vi "Main.vi"() -> ()   [LabVIEW 2019]
doc: "Use this template to build a simple state machine design pattern. Each state executes code and determines which state to transition to."
uses:
  <vilib>/Utility/file.llb/Write Delimited Spreadsheet (string).vi
panel:
  out "error out 2":errorcluster
  out "error out":errorcluster
  in  "Focus":bool
  in  "Start":bool
  in  "File Open":bool
  out "GPS Data":string[][](table)
  in  "Add":bool
  out "GPS Status":bool
  out "Image folder":path caption="Path"
  out "Statusbar":string="Idle"
  out "Build Version":string="Idle" caption="V"
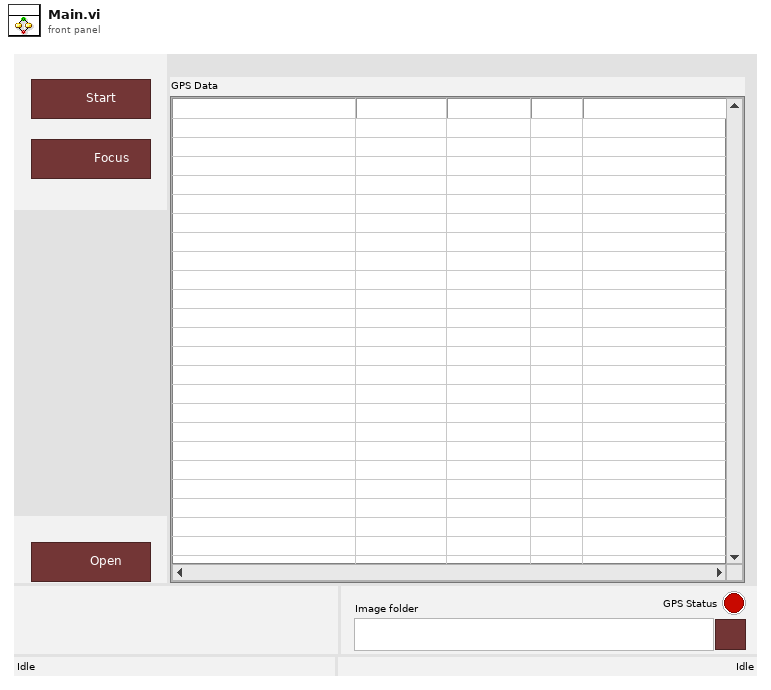
[diagram p1: front panel]
types:
  T1 = enum32{"Invalid", "Standard", "Closed", "Hidden", "Minimized", "Maximized"}
  T2 = enum32{"invalid app kind", "Development System", "Run Time System", "Student Edition", "Embedded LabVIEW", "Evaluation", "Custom"}
  T3 = typedef "System Data.ctl" = cluster{"System":cluster{"Active":bool, "Exit":bool, "Command wait":string, "Status_Time":i32, "Time_GPS":i32}, "Stepper Motor":T4, "Camera Data":T5, "Core":cluster{"Close Panel on Exit?":bool, "Current VI Reference":refnum<vi>}}
  T4 = typedef "Stepper Data.ctl" = cluster{"Connection Reference":refnum<visa-resource-name>, "Valid Connection":bool, "Speed":i32}
  T5 = typedef "Camera Data.ctl" = cluster{"Image path":path, "Filenames":string[], "Filenames queue":string[]}
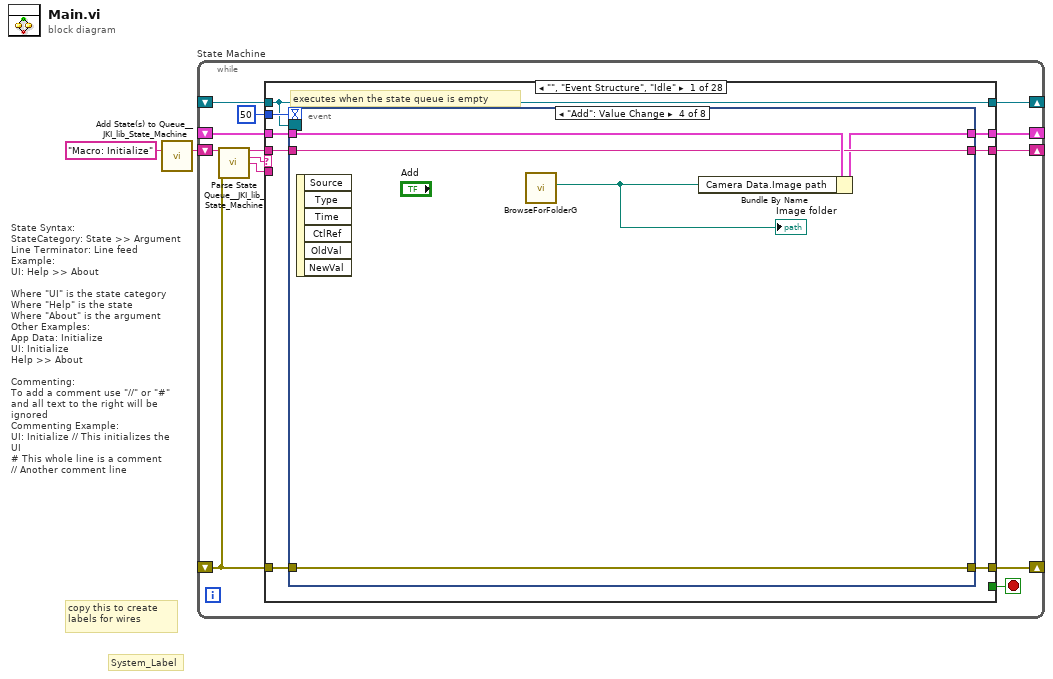
[diagram p0: block diagram]
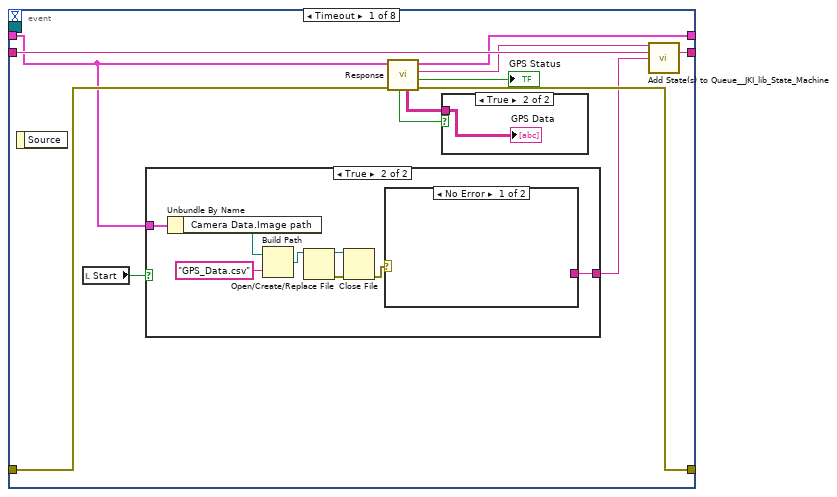
[diagram p2: hidden frame]
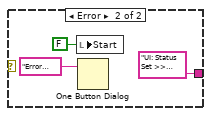
[diagram p5: hidden frame]
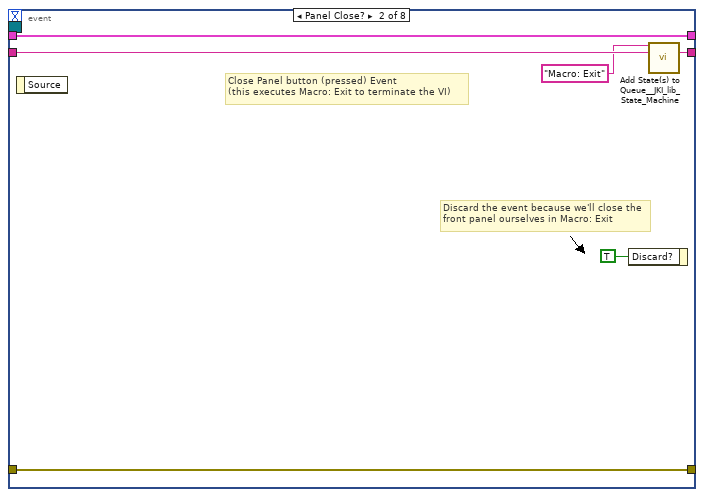
[diagram p6: hidden frame]
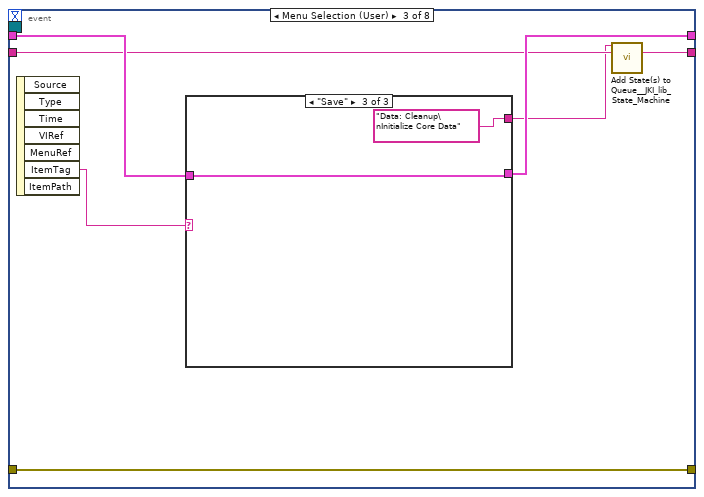
[diagram p7: hidden frame]
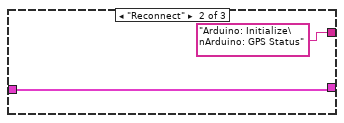
[diagram p9: hidden frame]
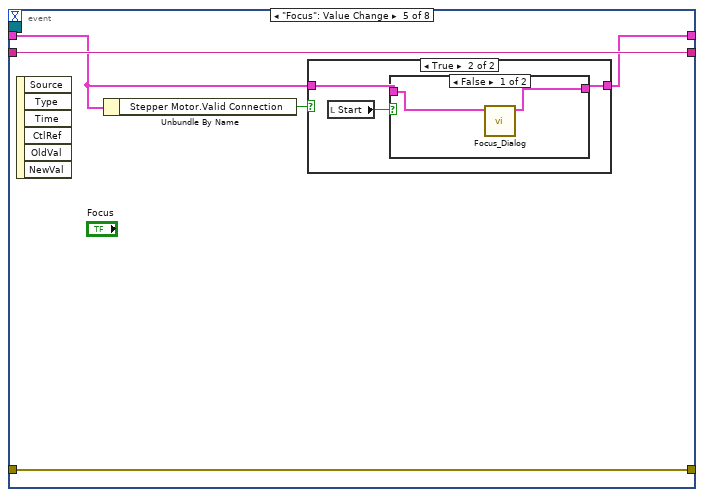
[diagram p10: hidden frame]
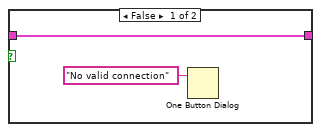
[diagram p11: hidden frame]
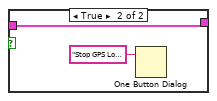
[diagram p12: hidden frame]
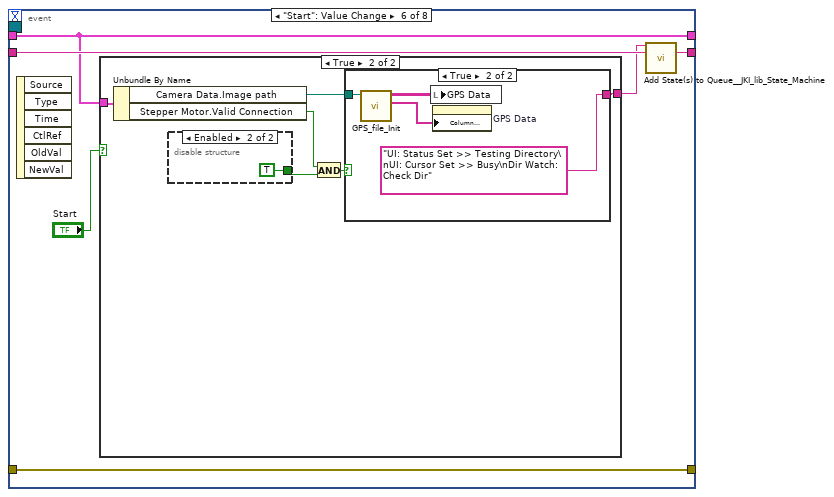
[diagram p13: hidden frame]
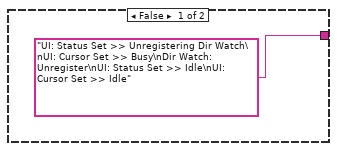
[diagram p14: hidden frame]
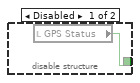
[diagram p15: hidden frame]
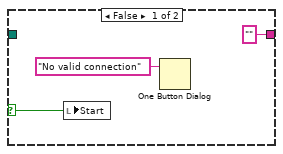
[diagram p16: hidden frame]
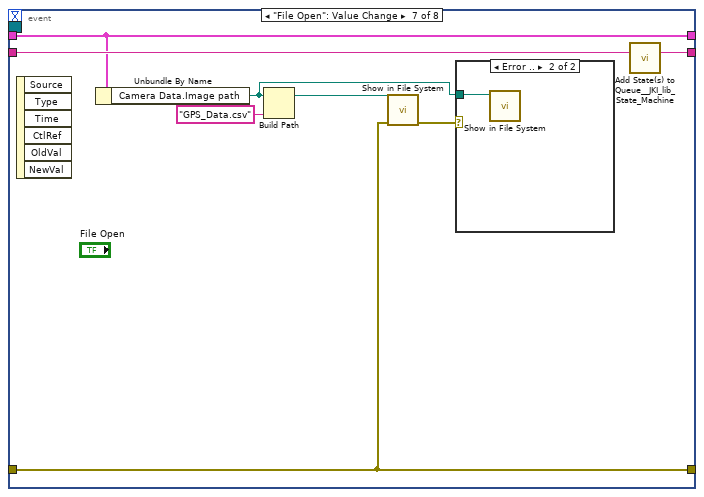
[diagram p17: hidden frame]
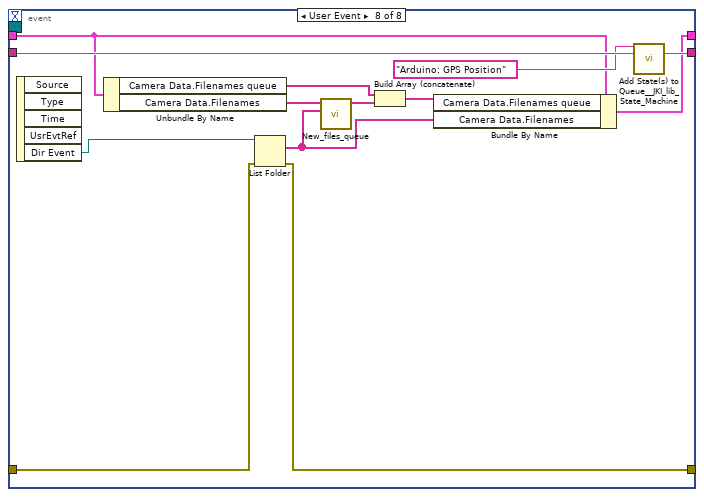
[diagram p19: hidden frame]
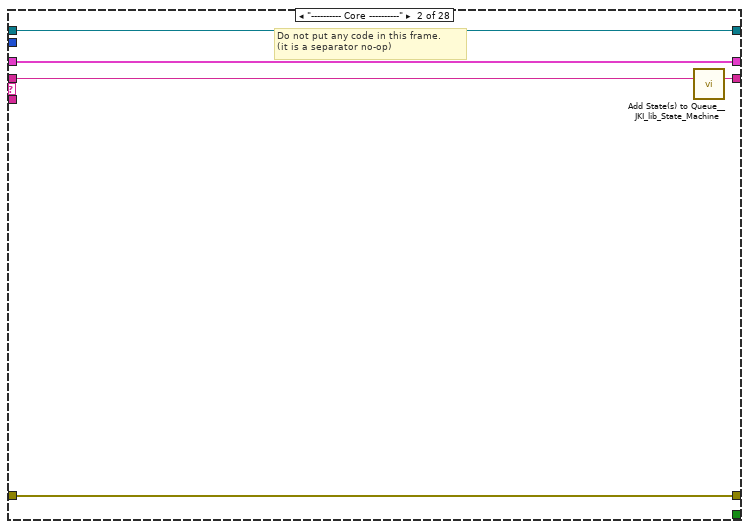
[diagram p20: hidden frame]
diagram:
  # "State Syntax:\nStateCategory: State >> Argument\nLine Terminator: Line feed\nExample:\nUI: Help >> About\n\nWhere \"UI\" is the state category\nWhere \"Help\" is the state\nWhere \"About\" is the argument\nOther Examples:\nApp Data: Initialize\nUI: Initialize\nHelp >> About\n\nCommenting:\nTo add a comment use \"//\" or \"#\" and all text to the right will be ignored\nCommenting Example:\nUI: Initialize // This initializes the UI\n# This whole line is a comment\n// Another comment line"
  # "copy this to create labels for wires"
  # "System_Label"
  n1 = call <vilib>:"Add State(s) to Queue__JKI_lib_State_Machine.vi"("State(s) in (\"\")"="Macro: Initialize") -> ("States Out"=w2:string)  [unwired: 14 in]
  n2 = while "State Machine" {
    shift-right: [w8] -> _
    shift-left: _ -> [w7]
    shift-right: [w11] -> _
    shift-left: _ -> [w5]
    shift-right: [w10] -> _
    shift-left: w2 -> [w12]
    shift-right: [w4] -> _
    shift-left: _ -> [w3]
    stop <- w9 stop-if-true
    n3 = call <vilib>:"Parse State Queue__JKI_lib_State_Machine.vi"("State Queue"=w12, "Error In (no error)"=w5) -> ("Remaining States"=w14:string, "Current State"=w15:string, "Arguments"=w13:string)  [unwired: 11 in]
    n4 = case shown="\"\", \"Event Structure\", \"Idle\"" w15 {
      selector: w15 -> [_ _ w135 _ _ _ _ _ _ _ _ _ _ _ _ _ _ _ _ _ _ _ _ _ _ _ _ _]
      tunnel: w14 -> [w23 w133 w139 w159 w168 w174 w179 w191 w198 w204 w209 w216 w223 w233 w241 w311 w317 w331 w336 w342 w349 w356 w363 w369 w376 w382 w391 w410]
      tunnel: w13 -> [_ _ _ _ _ _ _ _ _ _ _ _ w218 w229 w238 _ _ _ _ _ _ _ _ _ _ _ _ _]
      tunnel: w7 -> [w21 w130 w137 w152 w165 w172 w176 _ w192 w201 w206 w213 w221 w231 w234 w308 w314 w328 w333 w338 w346 w353 w359 w366 w374 w380 w388 w400]
      tunnel: [w20 w131 w141 w156 errorcluster {"status"=FALSE, "code"=0, "source"=""} ("error out") w171 w177 w189 w194 w200 w207 w210 w219 w228 w236 w309 w315 w329 w334 w340 w344 w350 w361 w367 w370 w379 w389 w408] -> w11
      tunnel: w5 -> [w19 w131 w140 w156 w160 w171 w177 w189 w193 w200 w207 w210 w220 w228 w239 w309 w315 w329 w334 w340 w345 w351 w361 w367 w373 w378 w389 w408]
      tunnel: [w22 w132 w138 w158 w167 w173 w178 w190 w197 w203 w208 w215 w222 w232 w240 w310 w316 w330 w335 w341 w348 w355 w362 w368 w375 w381 w390 w409] -> w10
      tunnel: [_ _ _ _ _ TRUE _ _ _ _ _ _ _ _ _ _ _ _ _ _ _ _ _ _ _ _ _ _] -> w9
      tunnel: [w18 w130 w137 w157 w163 w172 w176 w187 w192 w201 w206 w213 w221 w231 w234 w308 w314 w324 w333 w337 w343 w352 w359 w366 w371 w380 w387 w400] -> w8
      tunnel: 50 ("Timeout") -> [w17 _ _ _ _ _ _ _ _ _ _ _ _ _ _ _ _ _ _ _ _ _ _ _ _ _ _ _]
      tunnel: [w16 w129 w134 w146 w164 w170 w175 w188 w195 w202 w205 w214 w217 w230 w237 w307 w312 w322 w332 w339 w347 w354 w360 w365 w372 w377 w384 w406] -> w4
      tunnel: w3 -> [w16 w129 w134 w146 w164 w170 w175 w188 w195 w202 w205 w214 w217 w230 w237 w307 w312 w322 w332 w339 w347 w354 w360 w365 _ w377 w384 w406]
      frame "", "Event Structure", "Idle" {
        # "executes when the state queue is empty"
        n5 = event shown="[3] \"Add\": Value Change" {
          selector: w16 -> [_ _ _ _ _ _ _ _]
          dyn-events: _ -> [_ _ _ _ _ _ _ _]
          timeout: w17 -> [_ _ _ _ _ _ _ _]
          tunnel: w23 -> [w35 w53 w56 w69 w75 w89 w114 w125]
          tunnel: [w34 w52 w55 w69 w75 w88 w113 w126] -> w22
          tunnel: w21 -> [w27 w50 w58 w70 w72 w85 w112 w122]
          tunnel: [w29 w51 w60 w68 w74 w90 w107 w116] -> w20
          tunnel: w19 -> [w33 w51 w60 w68 w74 w90 w107 w127]
          tunnel: [w32 w50 w57 w67 w73 w85 w112 w120] -> w18
          event Timeout {
            n6 = event-data() -> ()  [unwired: 1 in, 1 out]
            n7 = local read "Start"() -> (w28:bool)
            n8 = case shown="True" w28 {
              tunnel: w27 -> [_ w44]
              tunnel: [_ w41] -> w26
              frame False {
              }
              frame True {
                n9 = Unbundle By Name(w44) -> ("Camera Data.Image path"=w42:path)
                n10 = Build Path(base path=w42, name or relative path="GPS_Data.csv") -> (appended path=w38:path)
                n11 = Open/Create/Replace File(file path (use dialog)=w38) -> (refnum out=w40:refnum<file>, error out=w39:errorcluster)  [unwired: 5 in, 1 out]
                n12 = Close File(refnum=w40, error in=w39) -> (error out=w37:errorcluster)  [unwired: 1 out]
                n13 = case shown="No Error" w37 {
                  tunnel: [_ "UI: Status Set >> Unregistering Dir Watch\nUI: Cursor Set >> Busy\nDir Watch: Unregister\nUI: Status Set >> Idle\nUI: Cursor Set >> Idle"] -> w41
                  frame No Error {
                  }
                  frame Error {
                    n14 = local write "Start"(FALSE ("Start")) -> ()
                    n15 = One Button Dialog(message="Error accessing GPS file\n\nClose file if open") -> ()  [unwired: 1 in, 1 out]
                  }
                }
              }
            }
            n16 = call "Response.vi"("error in"=w33, "System Data"=w27) -> ("error out"=w29:errorcluster, "GPS Status"=→"GPS Status":bool, "next state"=w31:string, "System Data out"=w32:T3, "Data"=w24:string[][], "NewData"=w25:bool)  [unwired: 4 in]
            n17 = case shown="True" w25 {
              tunnel: w24 -> [_ w36]
              frame False {
              }
              frame True {
                "GPS Data" <- w36
              }
            }
            n18 = call <vilib>:"Add State(s) to Queue__JKI_lib_State_Machine.vi"("State(s) in Front (\"\")"=w31, "State(s) in (\"\")"=w35, "State(s) at Back (\"\")"=w26) -> ("States Out"=w34:string)  [unwired: 12 in]
          }
          event Panel Close? {
            # "Discard the event because we'll close the front panel ourselves in Macro: Exit"
            # "Close Panel button (pressed) Event\n(this executes Macro: Exit to terminate the VI)"
            n19 = event-data() -> ()  [unwired: 1 in, 1 out]
            n20 = event-data("Discard?"=TRUE) -> ()  [unwired: 1 in, 1 out]
            n21 = call <vilib>:"Add State(s) to Queue__JKI_lib_State_Machine.vi"("State(s) in Front (\"\")"="Macro: Exit", "State(s) in (\"\")"=w53) -> ("States Out"=w52:string)  [unwired: 13 in]
          }
          event Menu Selection (User) {
            n22 = event-data() -> ("ItemTag"=w59:string)  [unwired: 1 in, 6 out]
            n23 = case shown="\"Save\"" w59 {
              tunnel: w58 -> [w61 w63 w65]
              tunnel: [w61 w63 w65] -> w57
              tunnel: [_ "Arduino: Initialize\nArduino: GPS Status" "Data: Cleanup\nInitialize Core Data"] -> w54
              frame "False", Default {
              }
              frame "Reconnect" {
              }
              frame "Save" {
              }
            }
            n24 = call <vilib>:"Add State(s) to Queue__JKI_lib_State_Machine.vi"("State(s) in Front (\"\")"=w54, "State(s) in (\"\")"=w56) -> ("States Out"=w55:string)  [unwired: 13 in]
          }
          event "Add": Value Change {
            n25 = event-data() -> ()  [unwired: 1 in, 6 out]
            n26 = call "BrowseForFolderG.vi"() -> ("Selected Path"=w66:path)  [unwired: 8 in, 3 out]
            "Image folder" <- w66
            n27 = Bundle By Name(cluster=w70, "Camera Data.Image path"=w66) -> (w67:T3)
          }
          event "Focus": Value Change {
            n28 = event-data() -> ()  [unwired: 1 in, 6 out]
            n29 = Unbundle By Name(w72) -> ("Stepper Motor.Valid Connection"=w71:bool)
            n30 = case shown="True" w71 {
              tunnel: [w77 w80] -> w73
              tunnel: w72 -> [w77 w79]
              frame False {
                n31 = One Button Dialog(message="No valid connection") -> ()  [unwired: 1 in, 1 out]
              }
              frame True {
                n32 = local read "Start"() -> (w78:bool)
                n33 = case shown="False" w78 {
                  tunnel: [w82 w84] -> w80
                  tunnel: w79 -> [w81 w84]
                  frame False {
                    n34 = call "Focus_Dialog.vi"("System Data"=w81) -> ("System Data out"=w82:T3)  [unwired: 10 in]
                  }
                  frame True {
                    n35 = One Button Dialog(message="Stop GPS Log before focusing") -> ()  [unwired: 1 in, 1 out]
                  }
                }
              }
            }
          }
          event "Start": Value Change {
            n36 = event-data() -> ()  [unwired: 1 in, 6 out]
            n37 = case shown="True" "Start" {
              tunnel: ["UI: Status Set >> Unregistering Dir Watch\nUI: Cursor Set >> Busy\nDir Watch: Unregister\nUI: Status Set >> Idle\nUI: Cursor Set >> Idle" w97] -> w87
              tunnel: w85 -> [_ w92]
              frame False {
              }
              frame True {
                n38 = Unbundle By Name(w92) -> ("Camera Data.Image path"=w96:path, "Stepper Motor.Valid Connection"=w95:bool)
                n39 = disable-structure shown="Enabled" {
                  disable-tunnel: [w98 TRUE ("GPS Status")] -> w93
                  frame Disabled {
                    n40 = local read "GPS Status"() -> (w98:bool)
                  }
                  frame Enabled {
                  }
                }
                n41 = And(x=w95, y=w93) -> (x .and. y?=w94:bool)
                n42 = case shown="True" w94 {
                  selector: w94 -> [w100 _]
                  tunnel: ["" "UI: Status Set >> Testing Directory\nUI: Cursor Set >> Busy\nDir Watch: Check Dir"] -> w97
                  tunnel: w96 -> [_ w105]
                  frame False {
                    n43 = local write "Start"(w100) -> ()
                    n44 = One Button Dialog(message="No valid connection") -> ()  [unwired: 1 in, 1 out]
                  }
                  frame True {
                    n45 = call "GPS_file_Init.vi"("file path (dialog if empty)"=w105) -> ("Header"=w103:string[], "Data"=w104:string[][])  [unwired: 9 in]
                    n46 = local write "GPS Data"(w104) -> ()
                    n47 = property on="GPS Data" class="Tbl (strict)"("Column Headers[]"=w103) -> ()  [unwired: 2 in, 2 out]
                  }
                }
              }
            }
            n48 = call <vilib>:"Add State(s) to Queue__JKI_lib_State_Machine.vi"("State(s) in Front (\"\")"=w87, "State(s) in (\"\")"=w89) -> ("States Out"=w88:string)  [unwired: 13 in]
          }
          event "File Open": Value Change {
            n49 = event-data() -> ()  [unwired: 1 in, 6 out]
            n50 = Unbundle By Name(w112) -> ("Camera Data.Image path"=w108:path)
            n51 = Build Path(base path=w108, name or relative path="GPS_Data.csv") -> (appended path=w111:path)
            n52 = call <vilib>:"Show in File System.vi"("error in (no error)"=w107, "file or directory path"=w111) -> ("error out"=w109:errorcluster)  [unwired: 9 in]
            n53 = case shown="Error .." w109 {
              tunnel: w108 -> [_ w115]
              frame No Error {
              }
              frame Error {
                n54 = call <vilib>:"Show in File System.vi"("file or directory path"=w115) -> ()  [unwired: 10 in, 1 out]
              }
            }
            n55 = call <vilib>:"Add State(s) to Queue__JKI_lib_State_Machine.vi"("State(s) in (\"\")"=w114) -> ("States Out"=w113:string)  [unwired: 14 in]
          }
          event User Event {
            n56 = event-data() -> ("Dir Event"=w128:path)  [unwired: 1 in, 4 out]
            n57 = Unbundle By Name(w122) -> ("Camera Data.Filenames queue"=w117:string[], "Camera Data.Filenames"=w123:string[])
            n58 = List Folder(path=w128, error in=w127) -> (filenames=w119:string[], error out=w116:errorcluster)  [unwired: 2 in, 2 out]
            n59 = call "New_files_queue.vi"("filenames new"=w119, "filenames old"=w123) -> ("Filenames"=w121:string[])  [unwired: 9 in]
            n60 = Build Array (concatenate)(w117, w121) -> (w118:string[])
            n61 = Bundle By Name(cluster=w122, "Camera Data.Filenames queue"=w118, "Camera Data.Filenames"=w119) -> (w120:T3)
            n62 = call <vilib>:"Add State(s) to Queue__JKI_lib_State_Machine.vi"("State(s) in Front (\"\")"="Arduino: GPS Position" ("State(s) in Front (\"\")"), "State(s) in (\"\")"=w125) -> ("States Out"=w126:string)  [unwired: 13 in]
          }
        }
      }
      frame "---------- Core ----------" {
        # "Do not put any code in this frame.\n(it is a separator no-op)"
        n63 = call <vilib>:"Add State(s) to Queue__JKI_lib_State_Machine.vi"("State(s) in (\"\")"=w133) -> ("States Out"=w132:string)  [unwired: 14 in]
      }
      frame Default {
        w144 = 42 items=["No error", "Argument error", "Memory is full", "Out of zone", "End of file", "File already open", "Generic file I/O error", "File not found", "File permission error", "Disk is full", "Duplicate path", "Too many files open", "System feature not enabled", "Resource file not found", "Cannot add resource", "Resource not found", "Image not found", "Image memory error", "Pen does not exist", "Config type invalid", "Config token not found", "Config parse error", "Config memory error", "Bad external code format", "Bad external code offset", "External code not present", "Null window", "Destroy window error", "Null menu", "Print aborted", "Bad print record", "Print driver error", "Windows error during printing", "Memory error during printing", "Print dialog error", "Generic print error", "Invalid device refnum", "Device not found", "Device parameter error", "Device unit error", "Cannot open device", "Device call aborted", "Generic error", "Cancelled by user", "Object ID too low", "Object ID too high", "Object not in heap", "Unknown heap", "Unknown object (invalid DefProc)", "Unknown object (DefProc not in table)", "Message out of range", "Invalid (null) method", "Unknown message", "Manager call not supported", "Bad address", "Network operation in progress", "Network operation timed out", "Connection is busy", "Network attribute not supported", "Network error", "Address in use", "System out of memory", "Connection aborted", "Connection refused", "Not connected", "Already connected", "Connection closed", "Initialization error (interapplication manager)", "Bad occurrence", "Wait on unbound occurrence handler", "Occurrence queue overflow", "Datalog type conflict", "Unused", "Unrecognized type (interapplication manager)", "Memory corrupt", "Failed to make temporary DLL", "Old CIN version", "Drag socket not found", "Failed to load drop-object", "Failed to register OLE object", "Failed to release OLE object", "Format specifier type mismatch", "Unknown format specifier", "Too few format specifiers", "Too many format specifiers", "Scan failed", "Newer CIN version", "Error converting to variant", "Runtime menu error", "Password tampered", "Variant attribute not found", "Incompatible variant data type", "Event data is not available", "Event Store is not present", "Occurrence is not found", "Event Queue is not created", "Event info is not available", "Refnum passed is NULL", "Error retrieving Class GUID", "Error retrieving CoClass GUID", "Error retrieving TypeLib GUID.", "Bad built application magic bytes.", "Specific driver is different from the specific driver associated with the Logical Name.", "There is no session opened to the class driver.", "Max Error", "MAX - Error with config objects", "MAX - Error loading configuration", "MAX - Group not supported"]
        # "Current State"
        # "Do not delete, rename, or modify this frame.\n(this is used to capture unhandled states and typos)"
        # "Handle mistyped state name (developer tool)"
        n64 = Format Into String(format string="Software Exception: Unhandled State \"%s\"." ("message"), error in=w140, w135) -> (resulting string=w143:string, error out=w142:errorcluster)  [unwired: 1 in]
        n65 = call <vilib>:"Error Cluster From Error Code.vi"("show call chain? (False)"=TRUE, "error in (no error)"=w142, "error message (\"\")"=w143, "error code (0)"=w144) -> ("error out"=w141:errorcluster)  [unwired: 5 in]
        n66 = call <vilib>:"Add State(s) to Queue__JKI_lib_State_Machine.vi"("State(s) in (\"\")"=w139) -> ("States Out"=w138:string)  [unwired: 14 in]
      }
      frame "Initialize Core Data" {
        # "Do not delete, rename, or modify this frame.\n(this is used to determine panel behavior on exit)"
        # "originally closed?"
        # "exe?"
        # "If panel starts closed or is an EXE, then close it when we exit"
        n67 = property class="VI"() -> ("FP.State"=w149:T1)  [unwired: 2 in, 2 out]
        n68 = property class="App"() -> ("App.Kind"=w155:T2)  [unwired: 2 in, 2 out]
        n69 = control-ref of="Current VI Reference"() -> (w150:refnum<vi>)
        n70 = Equal?(x=w149, y=T1."Closed" ("Front Panel Window:State")) -> (x = y?=w147:bool)
        n71 = Equal?(x=w155, y=T2."Run Time System" ("Application:Kind")) -> (x = y?=w153:bool)
        n72 = Or(x=w147, y=w153) -> (x .or. y?=w151:bool)
        n73 = Bundle By Name(cluster=w152, "Core.Current VI Reference"=w150, "Core.Close Panel on Exit?"=w151) -> (w157:T3)
        n74 = call <vilib>:"Add State(s) to Queue__JKI_lib_State_Machine.vi"("State(s) in (\"\")"=w159) -> ("States Out"=w158:string)  [unwired: 14 in]
      }
      frame "Error Handler" {
        # "Handle any errors here.\nYou can also output any states to clean-up after errors occur"
        # "Clear error"
        n75 = call <vilib>:"Simple Error Handler.vi"("error in (no error)"=w160) -> ()  [unwired: 4 in, 5 out]
        n76 = Bundle By Name(cluster=w165, "Stepper Motor.Valid Connection"=FALSE) -> (w163:T3)
        n77 = call <vilib>:"Add State(s) to Queue__JKI_lib_State_Machine.vi"("State(s) in Front (\"\")"="Macro: Exit" ("State(s) in Front (\"\")"), "State(s) in (\"\")"=w168) -> ("States Out"=w167:string)  [unwired: 13 in]
      }
      frame "Exit" {
        # "Do not put any code in this frame.\n(No errors that occur here will be handled.)"
        n78 = call <vilib>:"Add State(s) to Queue__JKI_lib_State_Machine.vi"("State(s) in (\"\")"=w174) -> ("States Out"=w173:string)  [unwired: 14 in]
      }
      frame "---------- Data ----------" {
        # "Do not put any code in this frame.\n(It is a separator no-op. You can make a copy of this frame to create a new Data frame)"
        n79 = call <vilib>:"Add State(s) to Queue__JKI_lib_State_Machine.vi"("State(s) in (\"\")"=w179) -> ("States Out"=w178:string)  [unwired: 14 in]
      }
      frame "Data: Initialize" {
        # "Initialize the shift-register data, here.\n(data names are defined by what you wire into the bundle function)"
        n80 = control-ref of="This VI"() -> (w180:refnum<vi>)
        n81 = call "System_Data_Load.vi"() -> ("error out"=→"error out":errorcluster, "System Data"=w182:T3)  [unwired: 10 in]
        n82 = Bundle By Name(cluster=w182, "Core.Current VI Reference"=w180) -> (w181:T3)
        n83 = Bundle By Name(cluster=w181, "Stepper Motor.Valid Connection"=FALSE, "Camera Data.Filenames queue"=string[] [], "System.Time_GPS"=0) -> (w187:T3)
        n84 = call <vilib>:"Add State(s) to Queue__JKI_lib_State_Machine.vi"("State(s) in (\"\")"=w191) -> ("States Out"=w190:string)  [unwired: 14 in]
      }
      frame "Data: Cleanup" {
        # "Cleanup any data and references, here.\n(this is called automatically, by the Macro: Exit)"
        n85 = Unbundle By Name(w192) -> ("Core.Current VI Reference"=w196:refnum<vi>)
        n86 = Close Reference(reference=w196, error in (no error)=w193) -> (error out=w194:errorcluster)
        n87 = call <vilib>:"Add State(s) to Queue__JKI_lib_State_Machine.vi"("State(s) in (\"\")"=w198) -> ("States Out"=w197:string)  [unwired: 14 in]
      }
      frame "Data: Save" {
        # "Cleanup any data and references, here.\n(this is called automatically, by the Macro: Exit)"
        n88 = call "System_Data_Save.vi"("System Data"=w201) -> ("error out"=→"error out 2":errorcluster)  [unwired: 9 in, 1 out]
        n89 = call <vilib>:"Add State(s) to Queue__JKI_lib_State_Machine.vi"("State(s) in (\"\")"=w204) -> ("States Out"=w203:string)  [unwired: 14 in]
      }
      frame "---------- UI ----------" {
        # "Do not put any code in this frame.\n(It is a separator no-op. You can make a copy of this frame to create a new UI frame)"
        n90 = call <vilib>:"Add State(s) to Queue__JKI_lib_State_Machine.vi"("State(s) in (\"\")"=w209) -> ("States Out"=w208:string)  [unwired: 14 in]
      }
      frame "UI: Initialize" {
        # "Initialize the User Interface, here.\n(this is called automatically, by the Macro: Init)"
        n91 = Unbundle By Name(w213) -> ("Camera Data.Image path"=w212:path)
        n92 = local write "GPS Data"(string[][] [] ("Table Control")) -> ()
        n93 = local write "Image folder"(w212) -> ()
        n94 = call <vilib>:"Add State(s) to Queue__JKI_lib_State_Machine.vi"("State(s) in (\"\")"=w216) -> ("States Out"=w215:string)  [unwired: 14 in]
      }
      frame "UI: Cursor Set" {
        # "Argument"
        # "Set and Unset Cursor Busy.\n(Usage: \"UI: Cursor Set >> Busy|Idle\")"
        n95 = case shown="\"Busy\"" w218 {
          tunnel: w220 -> [w225 w227]
          tunnel: [w224 w226] -> w219
          frame "Idle", Default {
            n96 = call <vilib>:"Unset Busy.vi"("error in (no error)"=w225) -> ("error out"=w224:errorcluster)  [unwired: 10 in]
          }
          frame "Busy" {
            n97 = call <vilib>:"Set Busy.vi"("error in (no error)"=w227) -> ("error out"=w226:errorcluster)  [unwired: 9 in, 1 out]
          }
        }
        n98 = call <vilib>:"Add State(s) to Queue__JKI_lib_State_Machine.vi"("State(s) in (\"\")"=w223) -> ("States Out"=w222:string)  [unwired: 14 in]
      }
      frame "UI: Status Set" {
        # "Argument"
        # "Set statusbar status.\n(Usage: \"UI: Status Set >> Status\")"
        n99 = call <vilib>:"Add State(s) to Queue__JKI_lib_State_Machine.vi"("State(s) in (\"\")"=w233) -> ("States Out"=w232:string)  [unwired: 14 in]
        "Statusbar" <- w229
      }
      frame "UI: Front Panel State" {
        # "Argument"
        # "Set Front Panel Open or Closed\n(Usage: \"UI: Front Panel State >> Open|Close\")"
        n100 = Unbundle By Name(w234) -> ("Core.Current VI Reference"=w235:refnum<vi>)
        n101 = case shown="\"Open\", \"Standard\", Default" w238 {
          tunnel: w239 -> [w247 w262 w273 w286 w299]
          tunnel: [w249 w263 w275 w288 w301] -> w236
          tunnel: w235 -> [w248 w260 w274 w287 w300]
          frame "Open", "Standard", Default {
            w242 = T1."Standard" ("State")
            n102 = property class="VI"(reference=w248, error in=w247) -> (reference out=w245:refnum<vi>, error out=w246:errorcluster, "FP.State"=w244:T1)
            n103 = Not Equal?(x=w244, y=w242) -> (x != y?=w243:bool)
            n104 = case shown="True" w243 {
              tunnel: [w253 w255] -> w249
              tunnel: w246 -> [w252 w255]
              tunnel: w245 -> [w251 _]
              tunnel: w242 -> [w250 _]
              frame True {
                n105 = invoke class="VI" method="FP.Open"(reference=w251, error in=w252, "Activate"=TRUE, "State"=w250) -> (error out=w253:errorcluster)  [unwired: 1 in, 4 out]
              }
              frame False {
              }
            }
          }
          frame "Close", "Closed" {
            n106 = property class="VI"(reference=w260, error in=w262) -> (reference out=w259:refnum<vi>, error out=w261:errorcluster, "FP.State"=w257:T1)
            n107 = Not Equal?(x=w257, y=T1."Closed" ("Front Panel Window:State")) -> (x != y?=w256:bool)
            n108 = case shown="True" w256 {
              tunnel: [w264 w267] -> w263
              tunnel: w261 -> [w264 w266]
              tunnel: w259 -> [_ w265]
              frame False {
              }
              frame True {
                n109 = invoke class="VI" method="FP.Close"(reference=w265, error in=w266) -> (error out=w267:errorcluster)  [unwired: 1 in, 2 out]
              }
            }
          }
          frame "Hidden", "Hide" {
            w268 = T1."Hidden" ("State")
            n110 = property class="VI"(reference=w274, error in=w273) -> (reference out=w271:refnum<vi>, error out=w272:errorcluster, "FP.State"=w270:T1)
            n111 = Not Equal?(x=w270, y=w268) -> (x != y?=w269:bool)
            n112 = case shown="True" w269 {
              tunnel: [w279 w280] -> w275
              tunnel: w272 -> [w278 w280]
              tunnel: w271 -> [w277 _]
              tunnel: w268 -> [w276 _]
              frame True {
                n113 = invoke class="VI" method="FP.Open"(reference=w277, error in=w278, "State"=w276) -> (error out=w279:errorcluster)  [unwired: 2 in, 4 out]
              }
              frame False {
              }
            }
          }
          frame "Minimize", "Minimized" {
            w281 = T1."Minimized" ("State")
            n114 = property class="VI"(reference=w287, error in=w286) -> (reference out=w284:refnum<vi>, error out=w285:errorcluster, "FP.State"=w283:T1)
            n115 = Not Equal?(x=w283, y=w281) -> (x != y?=w282:bool)
            n116 = case shown="False" w282 {
              tunnel: [w292 w293] -> w288
              tunnel: w285 -> [w291 w293]
              tunnel: w284 -> [w290 _]
              tunnel: w281 -> [w289 _]
              frame True {
                n117 = invoke class="VI" method="FP.Open"(reference=w290, error in=w291, "State"=w289) -> (error out=w292:errorcluster)  [unwired: 2 in, 4 out]
              }
              frame False {
              }
            }
          }
          frame "Maximize", "Maximized" {
            w294 = T1."Maximized" ("State")
            n118 = property class="VI"(reference=w300, error in=w299) -> (reference out=w297:refnum<vi>, error out=w298:errorcluster, "FP.State"=w296:T1)
            n119 = Not Equal?(x=w296, y=w294) -> (x != y?=w295:bool)
            n120 = case shown="True" w295 {
              tunnel: [w305 w306] -> w301
              tunnel: w298 -> [w304 w306]
              tunnel: w297 -> [w303 _]
              tunnel: w294 -> [w302 _]
              frame True {
                n121 = invoke class="VI" method="FP.Open"(reference=w303, error in=w304, "State"=w302) -> (error out=w305:errorcluster)  [unwired: 2 in, 4 out]
              }
              frame False {
              }
            }
          }
        }
        n122 = call <vilib>:"Add State(s) to Queue__JKI_lib_State_Machine.vi"("State(s) in (\"\")"=w241) -> ("States Out"=w240:string)  [unwired: 14 in]
      }
      frame "---------- Macro ----------" {
        # "Do not put any code in this frame.\n(It is a separator no-op. You can make a copy of this frame to create a new Macro frame)"
        n123 = call <vilib>:"Add State(s) to Queue__JKI_lib_State_Machine.vi"("State(s) in (\"\")"=w311) -> ("States Out"=w310:string)  [unwired: 14 in]
      }
      frame "Macro: Initialize" {
        # "Initialization Macro\n(This is called once, when the VI starts)"
        n124 = call <vilib>:"Add State(s) to Queue__JKI_lib_State_Machine.vi"("State(s) in Front (\"\")"="UI: Cursor set >> Busy\nUI: Status set >> Initializing Data\nData: Initialize\nUI: Status set >> Initializing Core Data\nInitialize Core Data\nUI: Status set >> Saving Data\nData: Save\nUI: Status set >> Initializing UI\nUI: Initialize\nUI: Status set >> Connecting system\nArduino: Initialize\nUI: Front Panel State >> Open\nUI: Cursor set >> Idle\nUI: Status set >> Idle", "State(s) in (\"\")"=w317) -> ("States Out"=w316:string)  [unwired: 13 in]
      }
      frame "Macro: Exit" {
        # "Exit Macro\n(This is called once, when the VI exits)"
        n125 = Unbundle By Name(w328) -> ("Core.Close Panel on Exit?"=w327:bool)
        n126 = Bundle By Name(cluster=w328, "System.Exit"=TRUE) -> (w324:T3)
        n127 = Select(t="UI: Front Panel State >> Close", s=w327, f="") -> (s? t:f=w326:string)
        n128 = call <vilib>:"Add State(s) to Queue__JKI_lib_State_Machine.vi"("State(s) in Front (\"\")"="Data: Save\nArduino: Terminate", "State(s) in (\"\")"=w326, "State(s) at Back (\"\")"="Data: Cleanup\nExit" ("State(s) at Back (\"\")")) -> ("States Out"=w325:string)  [unwired: 12 in]
        n129 = call <vilib>:"Add State(s) to Queue__JKI_lib_State_Machine.vi"("State(s) in Front (\"\")"=w325, "State(s) in (\"\")"=w331) -> ("States Out"=w330:string)  [unwired: 13 in]
      }
      frame "---------- Arduino ----------" {
        # "Template Separator\n(You can make a copy of, or modify, this frame)"
        n130 = call <vilib>:"Add State(s) to Queue__JKI_lib_State_Machine.vi"("State(s) in (\"\")"=w336) -> ("States Out"=w335:string)  [unwired: 14 in]
      }
      frame "Arduino: Initialize" {
        # "Initialize Arduino.\n(Searches and initializes connection to the arduino)"
        n131 = call "Connecting.vi"("System Data"=w338) -> ("System Data out"=w337:T3)  [unwired: 10 in]
        n132 = call <vilib>:"Add State(s) to Queue__JKI_lib_State_Machine.vi"("State(s) in (\"\")"=w342) -> ("States Out"=w341:string)  [unwired: 14 in]
      }
      frame "Arduino: GPS Status" {
        # "Initialize the User Interface, here.\n(this is called automatically, by the Macro: Init)"
        n133 = call "Sat_Count.vi"("error in (no error)"=w345, "System Data"=w346) -> ("error out"=w344:errorcluster, "System Data out"=w343:T3)  [unwired: 8 in]
        n134 = call <vilib>:"Add State(s) to Queue__JKI_lib_State_Machine.vi"("State(s) in (\"\")"=w349) -> ("States Out"=w348:string)  [unwired: 14 in]
      }
      frame "Arduino: GPS Position" {
        # "Requests GPS Position\n(this is called automatically, by the Dir event)"
        n135 = call "GPS_Pos.vi"("error in (no error)"=w351, "System Data"=w353) -> ("error out"=w350:errorcluster, "System Data out"=w352:T3)  [unwired: 8 in]
        n136 = call <vilib>:"Add State(s) to Queue__JKI_lib_State_Machine.vi"("State(s) in (\"\")"=w356) -> ("States Out"=w355:string)  [unwired: 14 in]
      }
      frame "Arduino: Terminate" {
        # "Your code here.\n(You can make a copy of, or modify, this frame)"
        n137 = Unbundle By Name(w359) -> ("Stepper Motor.Connection Reference"=w357:refnum<visa-resource-name>, "Stepper Motor.Valid Connection"=w358:bool)
        n138 = case shown="True" w358 {
          tunnel: w357 -> [_ w364]
          frame False {
          }
          frame True {
            n139 = VISA Close(VISA resource name=w364) -> ()  [unwired: 1 in, 1 out]
          }
        }
        n140 = call <vilib>:"Add State(s) to Queue__JKI_lib_State_Machine.vi"("State(s) in (\"\")"=w363) -> ("States Out"=w362:string)  [unwired: 14 in]
      }
      frame "---------- Dir Watch ----------" {
        # "Template Separator\n(You can make a copy of, or modify, this frame)"
        n141 = call <vilib>:"Add State(s) to Queue__JKI_lib_State_Machine.vi"("State(s) in (\"\")"=w369) -> ("States Out"=w368:string)  [unwired: 14 in]
      }
      frame "Dir Watch: Event Register" {
        # "Your code here.\n(You can make a copy of, or modify, this frame)"
        n142 = call "Dir Watch.vi"("error in (no error)"=w373, "System Data"=w374) -> ("error out"=w370:errorcluster, "Event Refnum"=w372:refnum<event-registration>, "System Data out"=w371:T3)  [unwired: 7 in]
        n143 = call <vilib>:"Add State(s) to Queue__JKI_lib_State_Machine.vi"("State(s) in (\"\")"=w376) -> ("States Out"=w375:string)  [unwired: 14 in]
      }
      frame "Dir Watch: Unregister" {
        # "Unregister\nUnregisters event watcher"
        n144 = Unregister For Events(event registration refnum=w377, error in=w378) -> (error out=w379:errorcluster)
        n145 = call <vilib>:"Add State(s) to Queue__JKI_lib_State_Machine.vi"("State(s) in (\"\")"=w382) -> ("States Out"=w381:string)  [unwired: 14 in]
      }
      frame "Dir Watch: Check Dir" {
        # "Checks set directory access\n(You can make a copy of, or modify, this frame)"
        n146 = call "Dir Checker.vi"("System Data"=w388) -> ("error constant"=w386:errorcluster, "Image path"=w383:path, "System Data Out"=w387:T3)  [unwired: 8 in]
        n147 = local write "Image folder"(w383) -> ()
        n148 = case shown="Error .." w386 {
          tunnel: ["UI: Status Set >> Accessing GPS file\nDir Watch: Check File" ("State(s) in Front (\"\")") "UI: Cursor Set >> Idle\nUI: Status Set >> Idle" ("State(s) in Front (\"\")")] -> w385
          frame No Error {
          }
          frame Error {
            n149 = local write "Start"(FALSE ("Start")) -> ()
            n150 = One Button Dialog(message="Error starting GPS-Video link\n\nMissing video directory") -> ()  [unwired: 1 in, 1 out]
          }
        }
        n151 = call <vilib>:"Add State(s) to Queue__JKI_lib_State_Machine.vi"("State(s) in Front (\"\")"=w385, "State(s) in (\"\")"=w391) -> ("States Out"=w390:string)  [unwired: 13 in]
      }
      frame "Dir Watch: Check File" {
        # "Your code here.\n(You can make a copy of, or modify, this frame)"
        n152 = Unbundle By Name(w400) -> ("Camera Data.Image path"=w403:path)
        n153 = Build Path(base path=w403, name or relative path="GPS_Data.csv") -> (appended path=w398:path)
        n154 = call <vilib>:"Check if File or Folder Exists.vi"("path"=w398) -> ("file or folder exists?"=w399:bool, "dup path"=w396:path)  [unwired: 8 in, 1 out]
        n155 = case shown="False" w399 {
          tunnel: w396 -> [w415 w416]
          tunnel: [w411 w416] -> w397
          frame False {
            n156 = call-poly <vilib>:"Write Delimited Spreadsheet.vi"("file path (dialog if empty)"=w415, "1D data"=string[] ["img_name", "Longitude", "Latitude", "Altitude", "Time"], "append to file? (new file:F)"=FALSE, "delimiter (\\t)"=";" ("delimiter (\\t)")) -> ("new file path (Not A Path if cancelled)"=w411:path)  [unwired: 10 in, 1 out]
          }
          frame True {
          }
        }
        n157 = Open/Create/Replace File(file path (use dialog)=w397) -> (refnum out=w404:refnum<file>, error out=w405:errorcluster)  [unwired: 5 in, 1 out]
        n158 = Close File(refnum=w404, error in=w405) -> (error out=w401:errorcluster)  [unwired: 1 out]
        n159 = case shown="Error .." w401 {
          tunnel: ["UI: Status Set >> Setting up Dir Watch\nDir Watch: Event Register\nUI: Status Set >> System Active\nUI: Cursor Set >> Idle" ("State(s) in Front (\"\")") "UI: Cursor Set >> Idle\nUI: Status Set >> Idle" ("State(s) in Front (\"\")")] -> w407
          frame No Error {
          }
          frame Error {
            n160 = local write "Start"(FALSE ("Start")) -> ()
            n161 = One Button Dialog(message="Error accessing GPS file\n\nClose file if open") -> ()  [unwired: 1 in, 1 out]
          }
        }
        n162 = call <vilib>:"Add State(s) to Queue__JKI_lib_State_Machine.vi"("State(s) in Front (\"\")"=w407, "State(s) in (\"\")"=w410) -> ("States Out"=w409:string)  [unwired: 13 in]
      }
    }
  }
